vi "LSMcontroller_v56_from here for labview64bit.vi"() -> ()   [LabVIEW 2015] (continued)
                            n1346 = call "displayerrors.vi"() -> ("error IO"=w3777:errorcluster)
                            n1347 = call <vilib>:"General Error Handler.vi"("type of dialog (OK msg:1)"=w3776, "error in (no error)"=w3777) -> ("error out"=w3775:errorcluster)  [unwired: 9 in, 4 out]
                            n1348 = call <vilib>:"Clear Errors.vi"("error in (no error)"=w3775) -> ("error out"=w3774:errorcluster)  [unwired: 5 in, 1 out]
                            n1349 = call "seterrors.vi"("error IO"=w3774) -> ()
                          }
                          frame #8 {
                            w3787 = FALSE ("Value (Signaling)")
                            n1350 = local read "save\ndata"() -> (w3782:bool)
                            n1351 = call "2pparameters.vi"("command"="get") -> ("params out"=w3780:T12)  [unwired: 1 in]
                            n1352 = Unbundle By Name(w3780) -> ("auto OD"=w3778:bool)
                            n1353 = case shown="True" w3782 {
                              tunnel: w3781 -> [_ w3794]
                              frame False {
                              }
                              frame True {
                                n1354 = local read "filename prefix"() -> (w3795:string)
                                n1355 = call "closebinaryfiles.vi"() -> ()  [unwired: 12 in]
                                n1356 = local read "data dir"() -> (w3796:path)
                                n1357 = call "saveparams.vi"("timestamp"=w3794, "filename prefix in"=w3795, "data dir in"=w3796) -> ()  [unwired: 1 in]
                              }
                            }
                            n1358 = case shown="True" w3778 {
                              frame False {
                              }
                              frame True {
                                n1359 = call "configuration.vi"("command"="get") -> ("config out"=w3790:T13)  [unwired: 2 in, 1 out]
                                n1360 = call "2pparameters.vi"("command"="get") -> ("params out"=w3793:T12)  [unwired: 1 in]
                                n1361 = Unbundle By Name(w3790) -> ("point OD"=w3788:u16)
                                n1362 = Unbundle By Name(w3793) -> ("ODfilt"=w3789:u16)
                                n1363 = call "filterwheelcontrol_nothorlabslib.vi"("Current OD filt"=w3788, "New ODfilt"=w3789) -> ()  [unwired: 1 in]
                              }
                            }
                            n1364 = call "reset AO_DO_v3.vi"() -> ()  [unwired: 12 in]
                            n1365 = property on="Start" class="Bool (strict)"("Val(Sgnl)"=w3787) -> ()  [unwired: 2 in, 2 out]
                            n1366 = property on="Start" class="Bool (strict)"("Visible"=TRUE, "DisabledEnum"=T8."Enabled" ("Disabled")) -> ()  [unwired: 2 in, 2 out]
                            n1367 = property on="Stop" class="Bool (strict)"("Val(Sgnl)"=w3787) -> ()  [unwired: 2 in, 2 out]
                            n1368 = property on="Stop" class="Bool (strict)"("Visible"=FALSE, "DisabledEnum"=T8."Disabled" ("Disabled")) -> ()  [unwired: 2 in, 2 out]
                          }
                        }
                      }
                      frame "Line" {
                      }
                      frame "Resonant Ellipse", "freeform contour" {
                        n1369 = stacked-sequence {
                          seq-local: [w3811 _ _ _ _ _ _ _ _ _ _] -> [_ _ w4656 _ _ w4669 w4736 _ _ w5096 _]
                          seq-local: [w3810 _ _ _ _ _ _ _ _ _ _] -> [_ _ _ _ _ _ _ _ w4783 _ _]
                          seq-local: [w3809 _ _ _ _ _ _ _ _ _ _] -> [_ _ _ _ _ _ _ _ w4782 _ _]
                          seq-local: [w3808 _ _ _ _ _ _ _ _ _ _] -> [_ _ _ _ _ _ _ _ w4785 _ _]
                          seq-local: [w3807 _ _ _ _ _ _ _ _ _ _] -> [_ _ _ _ _ _ _ _ w4781 _ _]
                          seq-local: [w3806 _ _ _ _ _ _ _ _ _ _] -> [_ _ _ _ _ _ _ _ w4780 _ _]
                          seq-local: [w3805 _ _ _ _ _ _ _ _ _ _] -> [_ _ _ _ _ _ _ _ w4784 _ _]
                          seq-local: [w3804 _ _ _ _ _ _ _ _ _ _] -> [_ _ _ _ _ _ _ _ w4779 _ _]
                          seq-local: [w3803 _ _ _ _ _ _ _ _ _ _] -> [_ _ _ _ _ _ _ _ w4778 _ _]
                          seq-local: [w3802 _ _ _ _ _ _ _ _ _ _] -> [_ _ _ _ _ _ _ _ w4773 _ _]
                          seq-local: [w3801 _ _ _ _ _ _ _ _ _ _] -> [_ _ _ _ _ _ _ _ w4772 _ _]
                          seq-local: [w3800 _ _ _ _ _ _ _ _ _ _] -> [_ _ _ _ _ _ _ _ w4777 _ _]
                          seq-local: [w3799 _ _ _ _ _ _ _ _ _ _] -> [_ _ _ _ _ _ _ _ w4776 _ _]
                          seq-local: [w3798 _ _ _ _ _ _ _ _ _ _] -> [_ _ _ _ _ _ _ _ w4775 _ _]
                          seq-local: [w3797 _ _ _ _ _ _ _ _ _ _] -> [_ _ _ _ _ _ _ _ w4774 _ _]
                          frame #0 {
                            n1370 = local read "save\ndata"() -> (w3812:bool)
                            n1371 = Get Date/Time In Seconds() -> (seconds since 1Jan1904=w3813:timestamp)
                            n1372 = case shown="False" w3812 {
                              tunnel: w3813 -> [w3814 w3816]
                              tunnel: [w3814 w3815] -> w3811
                              frame False {
                              }
                              frame True {
                                n1373 = call "createdatafolder.vi"("timestamp in"=w3816) -> ("current data path"=w3817:path, "timestamp out"=w3815:timestamp)
                                n1374 = local write "data dir"(w3817) -> ()
                              }
                            }
                            n1375 = stacked-sequence {
                              tunnel: w3811 -> [w3823 _ _ _ _ _ _ _ _]
                              tunnel: [_ _ _ _ _ _ w3961 _ _] -> w3810
                              tunnel: [_ _ _ _ _ _ w3960 _ _] -> w3809
                              tunnel: [_ _ _ _ _ _ w3959 _ _] -> w3808
                              tunnel: [_ _ _ _ _ _ w3958 _ _] -> w3807
                              tunnel: [_ _ _ _ _ _ w3957 _ _] -> w3806
                              tunnel: [_ _ _ _ _ _ w3956 _ _] -> w3805
                              tunnel: [_ _ _ _ _ _ w3955 _ _] -> w3804
                              tunnel: [_ _ _ _ _ _ w3954 _ _] -> w3803
                              tunnel: [_ _ _ _ _ _ w3953 _ _] -> w3802
                              tunnel: [_ _ _ _ _ _ w3952 _ _] -> w3801
                              tunnel: [_ _ _ _ _ _ w3951 _ _] -> w3800
                              tunnel: [_ _ _ _ _ _ w3950 _ _] -> w3799
                              tunnel: [_ _ _ _ _ _ w3949 _ _] -> w3798
                              tunnel: [_ _ _ _ _ _ w3948 _ _] -> w3797
                              frame #0 {
                                n1376 = local write "graphtab"(T6."timetrace" ("graphtab")) -> ()
                                n1377 = local read "AI channels"() -> (w3827:i32[])
                                n1378 = local read "CI channels"() -> (w3828:i32[])
                                n1379 = property on="Stop" class="Bool (strict)"("Visible"=TRUE, "DisabledEnum"=T8."Enabled" ("Disabled")) -> ()  [unwired: 2 in, 2 out]
                                n1380 = property on="Start" class="Bool (strict)"("Visible"=FALSE, "DisabledEnum"=T8."Disabled and Grayed Out" ("Disabled")) -> ()  [unwired: 2 in, 2 out]
                                n1381 = Format Date/Time String(time format string (%c)="%Y%m%d", seconds (now)=w3823) -> (date/time string=w3822:string)  [unwired: 1 in]
                                n1382 = Format Date/Time String(time format string (%c)="%H%M%S", seconds (now)=w3823) -> (date/time string=w3821:string)  [unwired: 1 in]
                                n1383 = call "2pparameters.vi"("command"="get") -> ("params out"=w3830:T12)  [unwired: 1 in]
                                n1384 = Bundle By Name(cluster=w3830, "aAI"=w3827, "aCI"=w3828, "type"="Timetrace", "date"=w3822, "time"=w3821) -> (w3829:T12)
                                n1385 = call "X-array-databuffer.vi"("command"=enum16{"get", "set", "clear", "append"}."clear") -> ()  [unwired: 3 in, 2 out]
                                n1386 = call "Y-array-databuffer.vi"("command"=enum16{"get", "set", "clear", "append"}."clear") -> ()  [unwired: 3 in, 2 out]
                                n1387 = call "2pparameters.vi"("Params in"=w3829, "command"="set") -> ()  [unwired: 1 out]
                                n1388 = call "CH1-1D-temp.vi"("command"=enum16{"get", "set", "clear", "append"}."clear") -> ()  [unwired: 3 in, 2 out]
                                n1389 = call "CH2-1D-temp.vi"("command"=enum16{"get", "set", "clear", "append"}."clear") -> ()  [unwired: 3 in, 2 out]
                                n1390 = call "allAI-temp.vi"("command"=enum16{"get", "set", "clear", "append"}."clear") -> ()  [unwired: 3 in, 2 out]
                              }
                              frame #1 {
                                n1391 = call "configuration.vi"("command"="get") -> ("config out"=w3847:T13)  [unwired: 2 in, 1 out]
                                n1392 = Unbundle By Name(w3847) -> ("CI names"=w3848:string[], "AI names"=w3849:string[])
                                n1393 = call "2pparameters.vi"("command"="get") -> ("params out"=w3843:T12)  [unwired: 1 in]
                                n1394 = Unbundle By Name(w3843) -> ("aCI"=w3844:i32[], "aAI"=w3845:i32[])
                                n1395 = for {
                                tunnel: w3844 -> [w3859] mode=indexing
                                tunnel: w3848 -> [w3860]
                                tunnel: [w3858] -> w3850 mode=indexing
                                n1396 = Index Array(array=w3860, index=w3859) -> (element=w3858:string)
                                }
                                n1397 = for {
                                tunnel: w3845 -> [w3856] mode=indexing
                                tunnel: w3849 -> [w3857]
                                tunnel: [w3855] -> w3851 mode=indexing
                                n1398 = Index Array(array=w3857, index=w3856) -> (element=w3855:string)
                                }
                                n1399 = Build Array (concatenate)(w3850, w3851) -> (w3841:string[])
                                n1400 = for {
                                tunnel: w3841 -> [w3853] mode=indexing
                                tunnel: [w3852] -> w3840 mode=indexing
                                i -> [w3854]
                                n1401 = Bundle("String"=w3853, w3854) -> (w3852:cluster{"String":string, i32})  [unwired: 1 in]
                                }
                                n1402 = property on="graph1list" class="Ring (strict)"("StringsAndValues[]"=w3840) -> ()  [unwired: 2 in, 2 out]
                                n1403 = property on="graph2list" class="Ring (strict)"("StringsAndValues[]"=w3840) -> ()  [unwired: 2 in, 2 out]
                              }
                              frame #2 {
                                n1404 = call "2pparameters.vi"("command"="get") -> ("params out"=w3863:T12)  [unwired: 1 in]
                                n1405 = Unbundle By Name(w3863) -> ("auto OD"=w3861:bool, "autoshutter"=w3864:bool)
                                n1406 = case shown="True" w3861 {
                                frame False {
                                }
                                frame True {
                                n1407 = call "configuration.vi"("command"="get") -> ("config out"=w3867:T13)  [unwired: 2 in, 1 out]
                                n1408 = Unbundle By Name(w3867) -> ("contour OD"=w3868:u16)
                                n1409 = local read "ODfilt"() -> (w3865:u16)
                                n1410 = call "filterwheelcontrol_nothorlabslib.vi"("Current OD filt"=w3865, "New ODfilt"=w3868) -> ()  [unwired: 1 in]
                                }
                                }
                                n1411 = case shown="True" w3864 {
                                frame False {
                                }
                                frame True {
                                n1412 = call "shuttercontrol.vi"("command"="close") -> ()  [unwired: 1 in, 1 out]
                                }
                                }
                              }
                              frame #3 {
                                n1413 = local read "Vy-min draw"() -> (w3877:dbl)
                                n1414 = local read "Vy-max draw"() -> (w3876:dbl)
                                n1415 = local read "Vx-min draw"() -> (w3879:dbl)
                                n1416 = local read "Vx-max draw"() -> (w3878:dbl)
                                n1417 = local read "xpixels ref"() -> (w3875:i32)
                                n1418 = local read "ypixels ref"() -> (w3874:i32)
                                n1419 = local read "ROI Type"() -> (w3873:u16)
                                n1420 = local read "srateAODOtt"() -> (w3896:dbl)
                                n1421 = local read "# of frames"() -> (w3901:i32)
                                n1422 = local read "refreshtime"() -> (w3893:dbl)
                                n1423 = local read "Pel"() -> (w3872:dbl)
                                n1424 = local read "bin"() -> (w3899:dbl)
                                n1425 = local read "Override AI buffer"() -> (w3870:bool)
                                n1426 = local read "finite samples"() -> (w3908:bool)
                                n1427 = local read "srateAODOtt"() -> (w3895:dbl)
                                n1428 = local read "srateAODOtt"() -> (w3902:dbl)
                                n1429 = local read "continuous"() -> (w3907:bool)
                                n1430 = local read "Angle ref"() -> (w3880:dbl)
                                n1431 = local read "wavdet"() -> (w3909:bool)
                                n1432 = local read "Vx-ref"() -> (w3904:dbl)
                                n1433 = local read "Vy-ref"() -> (w3906:dbl)
                                n1434 = local read "avpp"() -> (w3905:i32)
                                n1435 = call "tt_timeandsamples.vi"("bin"=w3899, "refreshtime"=w3893, "srateAODOtt"=w3896, "tot#ofsamples"=w3901) -> ("refreshrate"=w3897:dbl, "refreshbuffer"=w3898:i32, "timetracecycles"=w3903:i32)  [unwired: 5 in]
                                n1436 = local read "bin"() -> (w3900:dbl)
                                n1437 = call "2pparameters.vi"("command"="get") -> ("params out"=w3912:T12)  [unwired: 1 in]
                                n1438 = Bundle By Name(cluster=w3912, "Drawing Mode"=w3873, "measpoints"=w3901, "tt_cycles"=w3903, "refreshbuffer"=w3898, "refreshrate"=w3897, "Vx-ref"=w3904, "Vy-ref"=w3906, "srate"=w3895, "finite"=w3908, "cont"=w3907, "wavdet"=w3909, "avpp"=w3905, "srateAODO"=w3902, "bufferAI"=w3898, "bin"=w3900, "Angle Img"=w3880, "Vxminref"=w3879, "Vxmaxref"=w3878, "Vyminref"=w3877, "Vymaxref"=w3876, "Xpixels Img"=w3875, "Ypixels Img"=w3874, "Pel"=w3872, "Vz-reset"=0.0, "AIoverride"=w3870) -> (w3910:T12)
                                n1439 = Reciprocal(x=w3897) -> (1/x=w3894:dbl)
                                n1440 = local write "refreshtime"(w3894) -> ()
                                n1441 = call "2pparameters.vi"("Params in"=w3910, "command"="set") -> ()  [unwired: 1 out]
                                n1442 = local read "Voltage Clamp"() -> (w3887:bool)
                                n1443 = local read "Current Clamp"() -> (w3888:bool)
                                n1444 = local read "Vholding (mV)"() -> (w3882:sgl)
                                n1445 = local read "CC_ICgain"() -> (w3886:dbl)
                                n1446 = local read "OCgain"() -> (w3883:sgl)
                                n1447 = local read "holdon"() -> (w3881:bool)
                                n1448 = call "patchparameters.vi"("command"="get") -> ("Params out"=w3890:T15)  [unwired: 1 in]
                                n1449 = Bundle By Name(cluster=w3890, "VC"=w3887, "CC"=w3888, "CC_icg (pA/mv)"=w3886, "VC_icg (mV/mV)"=10.0, "OCG (mV/pA)"=w3883, "OVG (mV/mV)"=0.1, "Vhold (mV)"=w3882, "holdon"=w3881) -> (w3889:T15)
                                n1450 = call "patchparameters.vi"("Params in"=w3889, "command"="set") -> ()  [unwired: 1 out]
                              }
                              frame #4 {
                                n1451 = call "2pparameters.vi"("command"="get") -> ("params out"=w3928:T12)  [unwired: 1 in]
                                n1452 = Unbundle By Name(w3928) -> ("srateAODO"=w3929:sgl, "Angle Img"=w3930:dbl, "Angle draw"=w3931:dbl, "Vxmaxref"=w3932:dbl, "Vxminref"=w3933:dbl, "Xpixels Img"=w3934:i32, "Ypixels Img"=w3935:i32, "Vymaxref"=w3936:dbl, "Vxminref"=w3937:dbl, "Drawing Mode"=w3938:u16, "Pel"=w3939:sgl)
                                n1453 = Add(x=w3930, y=w3931) -> (x+y=w3914:dbl)
                                n1454 = call "ROI-databuffer.vi"("command"=enum16{"get", "set", "clear", "append"}."get") -> ("array out"=w3922:cluster{"x":sgl, "y":sgl}[])  [unwired: 4 in]
                                n1455 = call "ScanningWaveform_v4.vi"("Vy-min"=w3937, "Vy-max"=w3936, "yPixels/tPixels"=w3935, "xPixels/rPixels"=w3934, "Vx-min"=w3933, "Vx-max"=w3932, "Drawing Mode"=w3938, "Angle"=w3914, "AOrate"=w3929, "Points"=w3922, "points in ellipse"=w3939) -> ("numPixels"=w3915:dbl, "Y-WaveArray"=w3916:dbl[], "P"=w3921:dbl, "X-WaveArray"=w3917:dbl[])  [unwired: 5 in]
                                n1456 = call "Y-array-databuffer.vi"("array in"=w3916, "command"=enum16{"get", "set", "clear", "append"}."set") -> ()  [unwired: 2 in, 2 out]
                                n1457 = call "X-array-databuffer.vi"("array in"=w3917, "command"=enum16{"get", "set", "clear", "append"}."set") -> ()  [unwired: 2 in, 2 out]
                                n1458 = call "2pparameters.vi"("command"="get") -> ("params out"=w3926:T12)  [unwired: 1 in]
                                n1459 = Bundle By Name(cluster=w3926, "P"=w3921, "sAOxy"=w3915, "Pel"=w3915) -> (w3918:T12)
                                n1460 = call "2pparameters.vi"("Params in"=w3918, "command"="set") -> ()  [unwired: 1 out]
                              }
                              frame #5 {
                                n1461 = call "X-array-databuffer.vi"("command"=enum16{"get", "set", "clear", "append"}."get") -> ("array out"=w3942:dbl[])  [unwired: 3 in, 1 out]
                                n1462 = call "Y-array-databuffer.vi"("command"=enum16{"get", "set", "clear", "append"}."get") -> ("array out"=w3945:dbl[])  [unwired: 3 in, 1 out]
                                n1463 = Index Array(array=w3942, index=0) -> (element=w3941:dbl)
                                n1464 = Index Array(array=w3945, index=0) -> (element=w3940:dbl)
                                n1465 = call "setposition.vi"("Vy"=w3940, "Vx"=w3941) -> ()  [unwired: 1 in]
                              }
                              frame #6 {
                                # "rem2Ps"
                                # "A2Ps"
                                # "Al"
                                # "Rl"
                                n1466 = stacked-sequence {
                                seq-local: [w3966 _ _ _ _ _ _ _ _ _ _] -> [_ w4078 _ w4139 _ w4225 _ _ _ _ _]
                                seq-local: [w3967 _ _ _ _ _ _ _ _ _ _] -> [_ w4079 w4089 _ w4194 _ _ _ _ _ _]
                                seq-local: [_ _ w4088 _ _ _ _ _ _ _ _] -> [_ _ _ _ w4188 _ _ _ _ _ _]
                                seq-local: [_ _ _ w4138 _ _ _ _ _ _ _] -> [_ _ _ _ _ w4224 _ _ _ _ _]
                                seq-local: [w3963 _ _ _ _ _ _ _ _ _ _] -> [_ w4075 _ _ _ _ _ _ w4410 w4478 _]
                                seq-local: [w3962 _ _ _ _ _ _ _ _ _ _] -> [_ w4074 _ _ _ _ _ _ w4411 w4479 _]
                                seq-local: [w3969 _ _ _ _ _ _ _ _ _ _] -> [_ _ _ _ _ _ w4263 _ w4409 w4477 _]
                                seq-local: [w3965 _ _ _ _ _ _ _ _ _ _] -> [_ w4073 _ _ _ _ w4262 w4330 _ _ _]
                                seq-local: [w3964 _ _ _ _ _ _ _ _ _ _] -> [_ w4072 _ _ _ _ w4261 w4329 _ _ _]
                                seq-local: [w3968 _ _ _ _ _ _ _ _ _ _] -> [_ _ _ _ _ _ w4260 w4328 _ _ _]
                                tunnel: [_ _ w4087 _ _ _ _ _ _ _ _] -> w3960
                                tunnel: [_ _ w4086 _ _ _ _ _ _ _ _] -> w3961
                                tunnel: [w3967 _ _ _ _ _ _ _ _ _ _] -> w3959
                                tunnel: [w3966 _ _ _ _ _ _ _ _ _ _] -> w3956
                                tunnel: [_ _ _ w4137 _ _ _ _ _ _ _] -> w3957
                                tunnel: [_ _ _ w4136 _ _ _ _ _ _ _] -> w3958
                                tunnel: [w3965 _ _ _ _ _ _ _ _ _ _] -> w3951
                                tunnel: [w3964 _ _ _ _ _ _ _ _ _ _] -> w3950
                                tunnel: [_ _ _ _ _ _ w4259 _ _ _ _] -> w3949
                                tunnel: [_ _ _ _ _ _ _ w4327 _ _ _] -> w3948
                                tunnel: [w3963 _ _ _ _ _ _ _ _ _ _] -> w3952
                                tunnel: [w3962 _ _ _ _ _ _ _ _ _ _] -> w3953
                                tunnel: [_ _ _ _ _ _ _ _ w4408 _ _] -> w3954
                                tunnel: [_ _ _ _ _ _ _ _ _ w4476 _] -> w3955
                                frame #0 {
                                # "for a next version, give ome thought to\nthe possibilit of intermittently updating the\nwaveforms. it will have to be a calculation\nbased on speed of CPU and program on the one hand\nand length of measurement on the other. but then it should be possible, in principle, to \nupdate the waveform on the fly and that way cut up a longer measurement in smaller parts."
                                n1467 = stacked-sequence {
                                tunnel: [w3970 _ _ _] -> w3967
                                tunnel: [_ w3982 _ _] -> w3966
                                tunnel: [_ _ _ w4039] -> w3962
                                tunnel: [_ _ _ w4038] -> w3963
                                tunnel: [_ _ _ w4037] -> w3969
                                tunnel: [_ _ w3997 _] -> w3965
                                tunnel: [_ _ w3996 _] -> w3964
                                tunnel: [_ _ w3995 _] -> w3968
                                frame #0 {
                                n1468 = call "configuration.vi"("command"="get") -> ("config out"=w3972:T13)  [unwired: 2 in, 1 out]
                                n1469 = Unbundle By Name(w3972) -> ("Voltage to Xgalvo"=w3971:i32)
                                n1470 = call "2pparameters.vi"("command"="get") -> ("params out"=w3976:T12)  [unwired: 1 in]
                                n1471 = in-place {
                                in-place-border: w3971 -> [w3981]
                                in-place-border: [w3978] -> w3970
                                n1472 = in-place-cluster #23(w3976) -> ("aAO"=w3980:u32[])
                                n1473 = call "add channel to active arrayv2.vi"("line array in"=w3980, "line to add"=w3981) -> ("line array out"=w3979:u32[], "addition"=w3978:bool)  [unwired: 1 out]
                                n1474 = in-place-cluster #23("aAO"=w3979) -> (w3974:T12)
                                }
                                n1475 = call "2pparameters.vi"("Params in"=w3974, "command"="set") -> ()  [unwired: 1 out]
                                }
                                frame #1 {
                                n1476 = call "configuration.vi"("command"="get") -> ("config out"=w3984:T13)  [unwired: 2 in, 1 out]
                                n1477 = Unbundle By Name(w3984) -> ("Voltage to Ygalvo"=w3983:i32)
                                n1478 = call "2pparameters.vi"("command"="get") -> ("params out"=w3988:T12)  [unwired: 1 in]
                                n1479 = in-place {
                                in-place-border: w3983 -> [w3993]
                                in-place-border: [w3990] -> w3982
                                n1480 = in-place-cluster #24(w3988) -> ("aAO"=w3992:u32[])
                                n1481 = call "add channel to active arrayv2.vi"("line array in"=w3992, "line to add"=w3993) -> ("line array out"=w3991:u32[], "addition"=w3990:bool)  [unwired: 1 out]
                                n1482 = in-place-cluster #24("aAO"=w3991) -> (w3986:T12)
                                }
                                n1483 = call "2pparameters.vi"("Params in"=w3986, "command"="set") -> ()  [unwired: 1 out]
                                }
                                frame #2 {
                                n1484 = call "2pparameters.vi"("command"="get") -> ("params out"=w3999:T12)  [unwired: 1 in]
                                n1485 = Unbundle By Name(w3999) -> ("autoshutter"=w3998:bool, "wavdet"=w3994:bool)
                                n1486 = case shown="False" w3998 {
                                tunnel: [w4004 w4024] -> w3997
                                tunnel: [w4003 FALSE ("removal")] -> w3996
                                tunnel: [w4002 w4022] -> w3995
                                tunnel: w3994 -> [w4001 _]
                                frame False {
                                n1487 = case shown="False" w4001 {
                                tunnel: [FALSE ("addition") FALSE ("addition")] -> w4004
                                tunnel: [w4006 FALSE ("removal")] -> w4003
                                tunnel: [w4005 _] -> w4002
                                frame False {
                                n1488 = call "configuration.vi"("command"="get") -> ("config out"=w4012:T13)  [unwired: 2 in, 1 out]
                                n1489 = Unbundle By Name(w4012) -> ("2P shutter"=w4009:i32)
                                n1490 = call "2pparameters.vi"("command"="get") -> ("params out"=w4010:T12)  [unwired: 1 in]
                                n1491 = in-place {
                                in-place-border: w4009 -> [w4019]
                                in-place-border: [w4016] -> w4006
                                in-place-border: [w4015] -> w4005
                                n1492 = in-place-cluster #25(w4010) -> ("aDO"=w4018:u32[])
                                n1493 = call "remove channel from active arrayv2.vi"("line array in"=w4018, "line to remove"=w4019) -> ("line array out"=w4017:u32[], "removal"=w4016:bool, "index"=w4015:i32)
                                n1494 = in-place-cluster #25("aDO"=w4017) -> (w4007:T12)
                                }
                                n1495 = call "2pparameters.vi"("Params in"=w4007, "command"="set") -> ()  [unwired: 1 out]
                                }
                                frame True {
                                }
                                }
                                }
                                frame True {
                                n1496 = call "configuration.vi"("command"="get") -> ("config out"=w4026:T13)  [unwired: 2 in, 1 out]
                                n1497 = call "2pparameters.vi"("command"="get") -> ("params out"=w4030:T12)  [unwired: 1 in]
                                n1498 = Unbundle By Name(w4026) -> ("2P shutter"=w4025:i32)
                                n1499 = in-place {
                                in-place-border: w4025 -> [w4036]
                                in-place-border: [w4033] -> w4024
                                in-place-border: [w4032] -> w4022
                                n1500 = in-place-cluster #26(w4030) -> ("aDO"=w4035:u32[])
                                n1501 = call "add channel to active arrayv2.vi"("line array in"=w4035, "line to add"=w4036) -> ("line array out"=w4034:u32[], "addition"=w4033:bool, "index"=w4032:i32)
                                n1502 = in-place-cluster #26("aDO"=w4034) -> (w4028:T12)
                                }
                                n1503 = call "2pparameters.vi"("Params in"=w4028, "command"="set") -> ()  [unwired: 1 out]
                                }
                                }
                                }
                                frame #3 {
                                n1504 = local read "Measurement"() -> (w4040:T5)
                                n1505 = To Unsigned Long Integer(number=w4040) -> (unsigned 32bit integer=w4041:u32)
                                n1506 = case shown="5..7" w4041 {
                                tunnel: [FALSE ("addition") w4059] -> w4039
                                tunnel: [w4044 FALSE ("removal")] -> w4038
                                tunnel: [w4042 w4057] -> w4037
                                frame 0..4, Default {
                                n1507 = call "configuration.vi"("command"="get") -> ("config out"=w4050:T13)  [unwired: 2 in, 1 out]
                                n1508 = Unbundle By Name(w4050) -> ("LT timestamp"=w4047:u32)
                                n1509 = call "2pparameters.vi"("command"="get") -> ("params out"=w4048:T12)  [unwired: 1 in]
                                n1510 = in-place {
                                in-place-border: w4047 -> [w4056]
                                in-place-border: [w4053] -> w4044
                                in-place-border: [w4052] -> w4042
                                n1511 = in-place-cluster #27(w4048) -> ("aDO"=w4055:u32[])
                                n1512 = call "remove channel from active arrayv2.vi"("line array in"=w4055, "line to remove"=w4056) -> ("line array out"=w4054:u32[], "removal"=w4053:bool, "index"=w4052:i32)
                                n1513 = in-place-cluster #27("aDO"=w4054) -> (w4045:T12)
                                }
                                n1514 = call "2pparameters.vi"("Params in"=w4045, "command"="set") -> ()  [unwired: 1 out]
                                }
                                frame 5..7 {
                                n1515 = call "configuration.vi"("command"="get") -> ("config out"=w4065:T13)  [unwired: 2 in, 1 out]
                                n1516 = Unbundle By Name(w4065) -> ("LT timestamp"=w4062:u32)
                                n1517 = call "2pparameters.vi"("command"="get") -> ("params out"=w4063:T12)  [unwired: 1 in]
                                n1518 = in-place {
                                in-place-border: w4062 -> [w4071]
                                in-place-border: [w4068] -> w4059
                                in-place-border: [w4067] -> w4057
                                n1519 = in-place-cluster #28(w4063) -> ("aDO"=w4070:u32[])
                                n1520 = call "add channel to active arrayv2.vi"("line array in"=w4070, "line to add"=w4071) -> ("line array out"=w4069:u32[], "addition"=w4068:bool, "index"=w4067:i32)
                                n1521 = in-place-cluster #28("aDO"=w4069) -> (w4060:T12)
                                }
                                n1522 = call "2pparameters.vi"("Params in"=w4060, "command"="set") -> ()  [unwired: 1 out]
                                }
                                }
                                }
                                }
                                }
                                frame #1 {
                                n1523 = Or(x=w4078, y=w4079) -> (x .or. y?=w4077:bool)
                                n1524 = case shown="True" w4077 {
                                frame False {
                                }
                                frame True {
                                # "update GUI"
                                n1525 = call "Used AO lines.vi"() -> ("used AO names"=w4083:string[], "used AO lines"=w4085:tag[])  [unwired: 2 in]
                                n1526 = control-ref of="Analog Lines Plot"() -> (w4084:refnum<vi>)
                                n1527 = local write "Analog Used Lines"(w4085) -> ()
                                n1528 = local write "Analog Used Names"(w4083) -> ()
                                n1529 = call "prepAOWaveplot.vi"("WaveformGraph in"=w4084, "Analog Used Names"=w4083) -> ()  [unwired: 1 in]
                                }
                                }
                                n1530 = Compound Arithmetic op=OR(w4075, w4074, w4073, w4072) -> (w4076:bool)
                                n1531 = case shown="True" w4076 {
                                frame False {
                                }
                                frame True {
                                n1532 = control-ref of="Digital Lines Plot"() -> (w4080:refnum<vi>)
                                n1533 = call "Used DO lines.vi"() -> ("used DO names"=w4081:string[], "used DO lines"=w4082:tag[])  [unwired: 2 in]
                                n1534 = local write "Digital Used Lines"(w4082) -> ()
                                n1535 = local write "Digital Used Names"(w4081) -> ()
                                n1536 = call "prepDOWaveplot.vi"("DigitalGraph in"=w4080, "used DO names"=w4081) -> ()  [unwired: 1 in]
                                }
                                }
                                }
                                frame #2 {
                                n1537 = case shown="False" w4089 {
                                tunnel: [w4092 w4118] -> w4088
                                tunnel: [w4091 w4116] -> w4087
                                tunnel: [w4090 _] -> w4086
                                frame False {
                                n1538 = stacked-sequence {
                                seq-local: [w4094 _] -> [_ w4109]
                                tunnel: [w4094 _] -> w4092
                                tunnel: [w4097 _] -> w4091
                                tunnel: [w4093 _] -> w4090
                                frame #0 {
                                n1539 = call "configuration.vi"("command"="get") -> ("config out"=w4105:T13)  [unwired: 2 in, 1 out]
                                n1540 = call "waveformparamsv2.vi"("command"="get") -> ("Params out"=w4099:T16)  [unwired: 4 in, 2 out]
                                n1541 = Unbundle By Name(w4105) -> ("Voltage to Xgalvo"=w4106:i32)
                                n1542 = call "2pparameters.vi"("command"="get") -> ("params out"=w4102:T12)  [unwired: 1 in]
                                n1543 = Unbundle By Name(w4099) -> ("AO parameters"=w4098:T17)
                                n1544 = Unbundle By Name(w4102) -> ("aAO"=w4103:u32[])
                                n1545 = call "waveformsAObuffer.vi"("command"="get") -> ("AO wf out"=w4095:waveform(dbl)[])  [unwired: 1 in]
                                n1546 = Search 1D Array(1D array=w4103, element=w4106) -> (index of element=w4094:i32)  [unwired: 1 in]
                                n1547 = Index Array(array=w4095, index=w4094) -> (element=w4093:waveform(dbl))
                                n1548 = Index Array(array=w4098, index=w4094) -> (element=w4097:T18)
                                }
                                frame #1 {
                                w4110 = 0.0 ("Step size (V)")
                                n1549 = local read "Meastab"() -> (w4108:enum32{"X-Y Image", "Linescan", "Timetrace"})
                                n1550 = case shown="\"X-Y Image\", Default" w4108 {
                                tunnel: [w4112 w4113] -> w4107
                                frame "X-Y Image", Default {
                                n1551 = local read "Sampling rate"() -> (w4112:dbl)
                                }
                                frame "Timetrace" {
                                n1552 = local read "srateAODOtt"() -> (w4113:dbl)
                                }
                                }
                                n1553 = call "replace AO XYwfparam.vi"("Baseline (V)"=w4110, "Start amplitude (V)"=w4110, "Cycles"=w4110, "Repeats"=w4110, "index of AO wave"=w4109, "Step size (V)"=w4110, "DC (%)"=w4110, "Sampling frequency (Hz)"=w4107, "Period (ms)"=w4110, "Cycle length (s)"=w4110, "Pulses"=w4110, "padding value"=w4110, "Matlab wave name"=path "xwave") -> ()  [unwired: 3 in]
                                }
                                }
                                }
                                frame True {
                                w4117 = 0.0 ("Repeats")
                                n1554 = local read "Meastab"() -> (w4115:enum32{"X-Y Image", "Linescan", "Timetrace"})
                                n1555 = case shown="\"X-Y Image\", Default" w4115 {
                                tunnel: [w4134 w4135] -> w4114
                                frame "X-Y Image", Default {
                                n1556 = local read "Sampling rate"() -> (w4134:dbl)
                                }
                                frame "Timetrace" {
                                n1557 = local read "srateAODOtt"() -> (w4135:dbl)
                                }
                                }
                                n1558 = call "2pparameters.vi"("command"="get") -> ("params out"=w4120:T12)  [unwired: 1 in]
                                n1559 = call "configuration.vi"("command"="get") -> ("config out"=w4123:T13)  [unwired: 2 in, 1 out]
                                n1560 = call "waveformparamsv2.vi"("command"="get") -> ("Params out"=w4131:T16)  [unwired: 4 in, 2 out]
                                n1561 = Unbundle By Name(w4123) -> ("Voltage to Xgalvo"=w4124:i32)
                                n1562 = Unbundle By Name(w4131) -> ("AO parameters"=w4128:T17)
                                n1563 = Unbundle By Name(w4120) -> ("aAO"=w4121:u32[])
                                n1564 = Search 1D Array(1D array=w4121, element=w4124) -> (index of element=w4118:i32)  [unwired: 1 in]
                                n1565 = Index Array(array=w4128, index=0) -> (element=w4129:T18)
                                n1566 = Bundle By Name(cluster=w4129, "AOtab"=-1.0 ("Repeats"), "Repeats"=w4117, "Cycles"=w4117, "Start amplitude (V)"=w4117, "Baseline (V)"=w4117, "Step size (V)"=w4117, "DC (%)"=w4117, "Sampling frequency (Hz)"=w4114, "Period (ms)"=w4117, "Offset (V)"=w4117, "Amplitude (V)"=w4117, "Frequency"=w4117, "Tri Repeats"=w4117, "phase shift (ms)"=w4117, "Pulses"=w4117, "Matlab wave file"=path "xwave", "padding value"=w4117) -> (w4116:T18)
                                n1567 = Build Array(w4116) -> (w4126:T17)
                                n1568 = call "waveformparamsv2.vi"("command"="add AO", "add AO"=w4126) -> ()  [unwired: 3 in, 3 out]
                                }
                                }
                                }
                                frame #3 {
                                n1569 = case shown="True" w4139 {
                                tunnel: [w4142 w4168] -> w4138
                                tunnel: [w4141 w4166] -> w4137
                                tunnel: [w4140 _] -> w4136
                                frame False {
                                n1570 = stacked-sequence {
                                seq-local: [w4144 _] -> [_ w4159]
                                tunnel: [w4144 _] -> w4142
                                tunnel: [w4147 _] -> w4141
                                tunnel: [w4143 _] -> w4140
                                frame #0 {
                                n1571 = call "configuration.vi"("command"="get") -> ("config out"=w4155:T13)  [unwired: 2 in, 1 out]
                                n1572 = call "waveformparamsv2.vi"("command"="get") -> ("Params out"=w4149:T16)  [unwired: 4 in, 2 out]
                                n1573 = Unbundle By Name(w4155) -> ("Voltage to Ygalvo"=w4156:i32)
                                n1574 = call "2pparameters.vi"("command"="get") -> ("params out"=w4152:T12)  [unwired: 1 in]
                                n1575 = Unbundle By Name(w4149) -> ("AO parameters"=w4148:T17)
                                n1576 = Unbundle By Name(w4152) -> ("aAO"=w4153:u32[])
                                n1577 = call "waveformsAObuffer.vi"("command"="get") -> ("AO wf out"=w4145:waveform(dbl)[])  [unwired: 1 in]
                                n1578 = Search 1D Array(1D array=w4153, element=w4156) -> (index of element=w4144:i32)  [unwired: 1 in]
                                n1579 = Index Array(array=w4145, index=w4144) -> (element=w4143:waveform(dbl))
                                n1580 = Index Array(array=w4148, index=w4144) -> (element=w4147:T18)
                                }
                                frame #1 {
                                w4160 = 0.0 ("Step size (V)")
                                n1581 = local read "Meastab"() -> (w4158:enum32{"X-Y Image", "Linescan", "Timetrace"})
                                n1582 = case shown="\"X-Y Image\", Default" w4158 {
                                tunnel: [w4162 w4163] -> w4157
                                frame "X-Y Image", Default {
                                n1583 = local read "Sampling rate"() -> (w4162:dbl)
                                }
                                frame "Timetrace" {
                                n1584 = local read "srateAODOtt"() -> (w4163:dbl)
                                }
                                }
                                n1585 = call "replace AO XYwfparam.vi"("Baseline (V)"=w4160, "Start amplitude (V)"=w4160, "Cycles"=w4160, "Repeats"=w4160, "index of AO wave"=w4159, "Step size (V)"=w4160, "DC (%)"=w4160, "Sampling frequency (Hz)"=w4157, "Period (ms)"=w4160, "Cycle length (s)"=w4160, "Pulses"=w4160, "padding value"=w4160, "Matlab wave name"=path "ywave") -> ()  [unwired: 3 in]
                                }
                                }
                                }
                                frame True {
                                w4167 = 0.0 ("Repeats")
                                n1586 = local read "Meastab"() -> (w4165:enum32{"X-Y Image", "Linescan", "Timetrace"})
                                n1587 = case shown="\"X-Y Image\", Default" w4165 {
                                tunnel: [w4184 w4185] -> w4164
                                frame "X-Y Image", Default {
                                n1588 = local read "Sampling rate"() -> (w4184:dbl)
                                }
                                frame "Timetrace" {
                                n1589 = local read "srateAODOtt"() -> (w4185:dbl)
                                }
                                }
                                n1590 = call "2pparameters.vi"("command"="get") -> ("params out"=w4170:T12)  [unwired: 1 in]
                                n1591 = call "configuration.vi"("command"="get") -> ("config out"=w4173:T13)  [unwired: 2 in, 1 out]
                                n1592 = call "waveformparamsv2.vi"("command"="get") -> ("Params out"=w4182:T16)  [unwired: 4 in, 2 out]
                                n1593 = Unbundle By Name(w4173) -> ("Voltage to Ygalvo"=w4174:i32)
                                n1594 = Unbundle By Name(w4182) -> ("AO parameters"=w4179:T17)
                                n1595 = Unbundle By Name(w4170) -> ("aAO"=w4171:u32[])
                                n1596 = Search 1D Array(1D array=w4171, element=w4174) -> (index of element=w4168:i32)  [unwired: 1 in]
                                n1597 = Index Array(array=w4179, index=0) -> (element=w4180:T18)
                                n1598 = Bundle By Name(cluster=w4180, "AOtab"=-1.0 ("Repeats"), "Repeats"=w4167, "Cycles"=w4167, "Start amplitude (V)"=w4167, "Baseline (V)"=w4167, "Step size (V)"=w4167, "DC (%)"=w4167, "Sampling frequency (Hz)"=w4164, "Period (ms)"=w4167, "Offset (V)"=w4167, "Amplitude (V)"=w4167, "Frequency"=w4167, "Tri Repeats"=w4167, "phase shift (ms)"=w4167, "Pulses"=w4167, "Matlab wave file"=path "ywave", "padding value"=w4167) -> (w4166:T18)
                                n1599 = Build Array(w4166) -> (w4177:T17)
                                n1600 = call "waveformparamsv2.vi"("command"="add AO", "add AO"=w4177) -> ()  [unwired: 3 in, 3 out]
                                }
                                }
                                }
                                frame #4 {
                                n1601 = call "2pparameters.vi"("command"="get") -> ("params out"=w4191:T12)  [unwired: 1 in]
                                n1602 = Unbundle By Name(w4191) -> ("wavdet"=w4190:bool, "Pel"=w4187:sgl, "refwfsize"=w4186:dbl, "srateAODO"=w4189:sgl)
                                n1603 = case shown="True" w4190 {
                                tunnel: [w4195 w4205] -> w4193
                                tunnel: w4189 -> [w4196 w4207]
                                tunnel: w4187 -> [_ w4203]
                                tunnel: w4186 -> [_ w4202]
                                frame False {
                                n1604 = call "X-array-databuffer.vi"("command"=enum16{"get", "set", "clear", "append"}."get") -> ("array out"=w4199:dbl[])  [unwired: 3 in, 1 out]
                                n1605 = Reciprocal(x=w4196) -> (1/x=w4197:sgl)
                                n1606 = Bundle By Name("Y"=w4199, "dt"=w4197) -> (w4195:waveform(dbl))  [unwired: 1 in]
                                }
                                frame True {
                                n1607 = To Double Precision Float(number=w4203) -> (double precision float=w4204:dbl)
                                n1608 = Divide(x=w4202, y=w4204) -> (x/y=w4201:dbl)
                                n1609 = Round Toward +Infinity(x=w4201) -> (ceil(x): smallest int >= x=w4200:dbl)
                                n1610 = call "X-array-databuffer.vi"("command"=enum16{"get", "set", "clear", "append"}."get") -> ("array out"=w4209:dbl[])  [unwired: 3 in, 1 out]
                                n1611 = Reciprocal(x=w4207) -> (1/x=w4208:sgl)
                                n1612 = for {
                                N: w4200 -> [_]
                                tunnel: w4209 -> [w4211]
                                tunnel: [w4211] -> w4206 mode=concatenating
                                }
                                n1613 = Bundle By Name("Y"=w4206, "dt"=w4208) -> (w4205:waveform(dbl))  [unwired: 1 in]
                                }
                                }
                                n1614 = case shown="True" w4194 {
                                tunnel: w4193 -> [w4213 w4219]
                                tunnel: w4188 -> [w4214 _]
                                frame False {
                                n1615 = call "waveformsAObuffer.vi"("command"="get") -> ("AO wf out"=w4217:waveform(dbl)[])  [unwired: 1 in]
                                n1616 = property on="refwf" class="Ring (strict)" props=["RingText", "Text"]() -> ()  [unwired: 2 in, 3 out]
                                n1617 = Replace Array Subset(array=w4217, new element=w4213, index=w4214) -> (w4212:waveform(dbl)[])
                                n1618 = call "waveformsAObuffer.vi"("AO wf in"=w4212, "command"="set") -> ()  [unwired: 1 out]
                                }
                                frame True {
                                n1619 = call "waveformsAObuffer.vi"("command"="get") -> ("AO wf out"=w4221:waveform(dbl)[])  [unwired: 1 in]
                                n1620 = Build Array (concatenate)(w4221, w4219) -> (w4218:waveform(dbl)[])
                                n1621 = call "waveformsAObuffer.vi"("AO wf in"=w4218, "command"="set") -> ()  [unwired: 1 out]
                                }
                                }
                                }
                                frame #5 {
                                n1622 = call "2pparameters.vi"("command"="get") -> ("params out"=w4233:T12)  [unwired: 1 in]
                                n1623 = Unbundle By Name(w4233) -> ("wavdet"=w4232:bool, "Pel"=w4230:sgl, "refwfsize"=w4231:dbl, "srateAODO"=w4226:sgl)
                                n1624 = To Double Precision Float(number=w4230) -> (double precision float=w4229:dbl)
                                n1625 = Divide(x=w4231, y=w4229) -> (x/y=w4228:dbl)
                                n1626 = Round Toward +Infinity(x=w4228) -> (ceil(x): smallest int >= x=w4227:dbl)
                                n1627 = case shown="True" w4232 {
                                tunnel: [w4237 w4243] -> w4223
                                tunnel: w4227 -> [_ w4240]
                                tunnel: w4226 -> [w4238 w4245]
                                frame False {
                                n1628 = call "Y-array-databuffer.vi"("command"=enum16{"get", "set", "clear", "append"}."get") -> ("array out"=w4235:dbl[])  [unwired: 3 in, 1 out]
                                n1629 = Reciprocal(x=w4238) -> (1/x=w4239:sgl)
                                n1630 = Bundle By Name("Y"=w4235, "dt"=w4239) -> (w4237:waveform(dbl))  [unwired: 1 in]
                                }
                                frame True {
                                n1631 = call "Y-array-databuffer.vi"("command"=enum16{"get", "set", "clear", "append"}."get") -> ("array out"=w4241:dbl[])  [unwired: 3 in, 1 out]
                                n1632 = Reciprocal(x=w4245) -> (1/x=w4246:sgl)
                                n1633 = for {
                                N: w4240 -> [_]
                                tunnel: w4241 -> [w4247]
                                tunnel: [w4247] -> w4244 mode=concatenating
                                }
                                n1634 = Bundle By Name("Y"=w4244, "dt"=w4246) -> (w4243:waveform(dbl))  [unwired: 1 in]
                                }
                                }
                                n1635 = case shown="False" w4225 {
                                tunnel: w4223 -> [w4250 w4255]
                                tunnel: w4224 -> [w4251 _]
                                frame False {
                                n1636 = call "waveformsAObuffer.vi"("command"="get") -> ("AO wf out"=w4253:waveform(dbl)[])  [unwired: 1 in]
                                n1637 = Replace Array Subset(array=w4253, new element=w4250, index=w4251) -> (w4248:waveform(dbl)[])
                                n1638 = call "waveformsAObuffer.vi"("AO wf in"=w4248, "command"="set") -> ()  [unwired: 1 out]
                                }
                                frame True {
                                n1639 = call "waveformsAObuffer.vi"("command"="get") -> ("AO wf out"=w4257:waveform(dbl)[])  [unwired: 1 in]
                                n1640 = Build Array (concatenate)(w4257, w4255) -> (w4254:waveform(dbl)[])
                                n1641 = call "waveformsAObuffer.vi"("AO wf in"=w4254, "command"="set") -> ()  [unwired: 1 out]
                                }
                                }
                                }
                                frame #6 {
                                n1642 = Build Array(w4262, w4261) -> (w4265:bool[])
                                n1643 = Boolean Array To Number(Boolean array=w4265) -> (number=w4264:u32)
                                n1644 = case shown="1" w4264 {
                                tunnel: w4263 -> [_ _ _ _]
                                tunnel: w4260 -> [_ w4288 _ w4301]
                                tunnel: [_ w4287 _ w4298] -> w4259
                                frame 1 {
                                w4275 = 0.0 ("DOtab")
                                n1645 = call "2pparameters.vi"("command"="get") -> ("params out"=w4272:T12)  [unwired: 1 in]
                                n1646 = call "waveformparamsv2.vi"("command"="get") -> ("Params out"=w4283:T16)  [unwired: 4 in, 2 out]
                                n1647 = Unbundle By Name(w4283) -> ("DO parameters"=w4281:T19)
                                n1648 = Unbundle By Name(w4272) -> ("srate"=w4268:sgl, "Pel"=w4271:sgl)
                                n1649 = To Double Precision Float(number=w4268) -> (double precision float=w4266:dbl)
                                n1650 = To Double Precision Float(number=w4268) -> (double precision float=w4267:dbl)
                                n1651 = To Double Precision Float(number=w4271) -> (double precision float=w4270:dbl)
                                n1652 = Divide(x=w4267, y=w4270) -> (x/y=w4269:dbl)
                                n1653 = Index Array(array=w4281, index=0) -> (element=w4280:T20)
                                n1654 = Bundle By Name(cluster=w4280, "Digital DC (%)"=100.0, "Digital phase"=w4275, "Digital Freq (Hz)"=w4269, "Sampling frequency (Hz)"=w4266, "Digital time offset (s)"=w4275, "padding value"=0.0, "matlab wave file"=path "2Pshutter", "DOtab"=0.0) -> (w4278:T20)
                                n1655 = Build Array(w4278) -> (w4277:T19)
                                n1656 = call "waveformparamsv2.vi"("command"="add DO", "add DO"=w4277) -> ()  [unwired: 3 in, 3 out]
                                }
                                frame 2 {
                                n1657 = call "waveformparamsv2.vi"("command"="get") -> ("Params out"=w4290:T16)  [unwired: 4 in, 2 out]
                                n1658 = in-place {
                                in-place-border: w4288 -> [w4294]
                                in-place-border: [w4293] -> w4287
                                n1659 = in-place-cluster #29(w4290) -> ("DO parameters"=w4296:T19)
                                n1660 = Delete From Array(array=w4296, length=1, index=w4294) -> (deleted portion=w4293:T19, array with subset deleted=w4295:T19)
                                n1661 = in-place-cluster #29("DO parameters"=w4295) -> (w4289:T16)
                                }
                                n1662 = call "waveformparamsv2.vi"("command"="set", "Params in"=w4289) -> ()  [unwired: 3 in, 3 out]
                                }
                                frame 3, Default {
                                }
                                frame 0 {
                                n1663 = call "2pparameters.vi"("command"="get") -> ("params out"=w4303:T12)  [unwired: 1 in]
                                n1664 = Unbundle By Name(w4303) -> ("wavdet"=w4300:bool, "autoshutter"=w4302:bool)
                                n1665 = case shown="True" w4302 {
                                tunnel: w4301 -> [_ w4307]
                                tunnel: w4300 -> [_ w4306]
                                tunnel: [_ w4305] -> w4299
                                frame False {
                                }
                                frame True {
                                n1666 = case shown="False" w4306 {
                                tunnel: w4307 -> [w4309 _]
                                tunnel: [w4308 _] -> w4305
                                frame False {
                                n1667 = stacked-sequence {
                                tunnel: w4309 -> [w4311 w4325]
                                tunnel: [w4310 _] -> w4308
                                frame #0 {
                                n1668 = call "waveformparamsv2.vi"("command"="get") -> ("Params out"=w4313:T16)  [unwired: 4 in, 2 out]
                                n1669 = Unbundle By Name(w4313) -> ("DO parameters"=w4312:T19)
                                n1670 = Index Array(array=w4312, index=w4311) -> (element=w4310:T20)
                                }
                                frame #1 {
                                w4324 = 0.0 ("padding value")
                                n1671 = call "2pparameters.vi"("command"="get") -> ("params out"=w4322:T12)  [unwired: 1 in]
                                n1672 = Unbundle By Name(w4322) -> ("srate"=w4319:sgl, "Pel"=w4321:sgl)
                                n1673 = To Double Precision Float(number=w4319) -> (double precision float=w4317:dbl)
                                n1674 = To Double Precision Float(number=w4319) -> (double precision float=w4318:dbl)
                                n1675 = To Double Precision Float(number=w4321) -> (double precision float=w4320:dbl)
                                n1676 = Divide(x=w4318, y=w4320) -> (x/y=w4316:dbl)
                                n1677 = call "replace DO wf param.vi"("Digital Freq (Hz)"=w4316, "Digital DC (%)"=100.0, "Digital phase"=w4324, "Sampling frequency (Hz)"=w4317, "Digital time offset (s)"=w4324, "index of DO wave"=w4325, "padding value"=w4324, "matlab wave file"=path "2Pshutter" ("matlab wave number")) -> ()  [unwired: 3 in]
                                }
                                }
                                }
                                frame True {
                                }
                                }
                                }
                                }
                                n1678 = Build Array(w4299) -> (w4298:T19)
                                }
                                }
                                }
                                frame #7 {
                                n1679 = Build Array(w4330, w4329) -> (w4332:bool[])
                                n1680 = Boolean Array To Number(Boolean array=w4332) -> (number=w4331:u32)
                                n1681 = case shown="0" w4331 {
                                tunnel: w4328 -> [_ w4374 _ w4381]
                                tunnel: [_ w4373 _ w4379] -> w4327
                                frame 1 {
                                n1682 = call "2pparameters.vi"("command"="get") -> ("params out"=w4339:T12)  [unwired: 1 in]
                                n1683 = Unbundle By Name(w4339) -> ("wavdet"=w4340:bool, "Pel"=w4342:sgl, "refwfsize"=w4343:dbl, "srateAODO"=w4341:sgl)
                                n1684 = call "waveformsDObuffer.vi"("command"="get") -> ("DO wf out"=w4335:digitalwaveform[])  [unwired: 1 in]
                                n1685 = case shown="False" w4340 {
                                tunnel: [w4348 w4358] -> w4337
                                tunnel: w4341 -> [w4353 w4369]
                                tunnel: w4342 -> [w4347 w4362]
                                tunnel: w4343 -> [_ w4366]
                                frame False {
                                w4351 = u16 0 items=["unsigned binary", "offset binary", "2's complement"] ("data format (offset binary)")
                                n1686 = Initialize Array(sgl 1.0, w4347) -> (w4344:sgl[])
                                n1687 = Reciprocal(x=w4353) -> (1/x=w4354:sgl)
                                n1688 = Bundle By Name("Y"=w4344, "dt"=w4354) -> (w4349:waveform(sgl))  [unwired: 1 in]
                                n1689 = call-poly <vilib>:"Analog to Digital.vi"("data format (offset binary)"=w4351, "compress digital (T)"=TRUE, "full-scale range (pk-pk)"=1.0, "resolution (16 bit)"=1, "analog waveform"=w4349) -> ("digital waveform"=w4348:digitalwaveform)  [unwired: 3 in, 3 out]
                                }
                                frame True {
                                w4361 = u16 0 items=["unsigned binary", "offset binary", "2's complement"] ("data format (offset binary)")
                                n1690 = To Double Precision Float(number=w4362) -> (double precision float=w4367:dbl)
                                n1691 = Initialize Array(sgl 1.0, w4362) -> (w4355:sgl[])
                                n1692 = Divide(x=w4366, y=w4367) -> (x/y=w4364:dbl)
                                n1693 = Round Toward +Infinity(x=w4364) -> (ceil(x): smallest int >= x=w4365:dbl)
                                n1694 = for {
                                N: w4365 -> [_]
                                tunnel: w4355 -> [w4371]
                                tunnel: [w4371] -> w4368 mode=concatenating
                                }
                                n1695 = Reciprocal(x=w4369) -> (1/x=w4370:sgl)
                                n1696 = Bundle By Name("Y"=w4368, "dt"=w4370) -> (w4359:waveform(sgl))  [unwired: 1 in]
                                n1697 = call-poly <vilib>:"Analog to Digital.vi"("data format (offset binary)"=w4361, "compress digital (T)"=TRUE, "full-scale range (pk-pk)"=1.0, "resolution (16 bit)"=1, "analog waveform"=w4359) -> ("digital waveform"=w4358:digitalwaveform)  [unwired: 3 in, 3 out]
                                }
                                }
                                n1698 = Build Array (concatenate)(w4335, w4337) -> (w4333:digitalwaveform[])
                                n1699 = call "waveformsDObuffer.vi"("DO wf in"=w4333, "command"="set") -> ()  [unwired: 1 out]
                                }
                                frame 2 {
                                n1700 = call "waveformsDObuffer.vi"("command"="get") -> ("DO wf out"=w4376:digitalwaveform[])  [unwired: 1 in]
                                n1701 = Delete From Array(array=w4376, length=1, index=w4374) -> (deleted portion=w4373:digitalwaveform[], array with subset deleted=w4372:digitalwaveform[])
                                n1702 = call "waveformsDObuffer.vi"("DO wf in"=w4372, "command"="set") -> ()  [unwired: 1 out]
                                }
                                frame 3, Default {
                                }
                                frame 0 {
                                n1703 = call "2pparameters.vi"("command"="get") -> ("params out"=w4383:T12)  [unwired: 1 in]
                                n1704 = Unbundle By Name(w4383) -> ("autoshutter"=w4382:bool, "wavdet"=w4380:bool)
                                n1705 = case shown="True" w4382 {
                                tunnel: w4381 -> [_ w4387]
                                tunnel: w4380 -> [_ w4386]
                                tunnel: [_ w4385] -> w4379
                                frame False {
                                }
                                frame True {
                                n1706 = case shown="False" w4386 {
                                tunnel: w4387 -> [w4391 _]
                                tunnel: [w4389 _] -> w4385
                                frame False {
                                w4398 = u16 0 items=["unsigned binary", "offset binary", "2's complement"] ("data format (offset binary)")
                                n1707 = call "2pparameters.vi"("command"="get") -> ("params out"=w4405:T12)  [unwired: 1 in]
                                n1708 = call "waveformsDObuffer.vi"("command"="get") -> ("DO wf out"=w4392:digitalwaveform[])  [unwired: 1 in]
                                n1709 = Unbundle By Name(w4405) -> ("Pel"=w4407:sgl, "srate"=w4406:sgl)
                                n1710 = Index Array(array=w4392, index=w4391) -> (element=w4390:digitalwaveform)
                                n1711 = Build Array(w4390) -> (w4389:digitalwaveform[])
                                n1712 = Initialize Array(sgl 1.0, w4407) -> (w4393:sgl[])
                                n1713 = Reciprocal(x=w4406) -> (1/x=w4400:sgl)
                                n1714 = Bundle By Name("Y"=w4393, "dt"=w4400) -> (w4396:waveform(sgl))  [unwired: 1 in]
                                n1715 = call-poly <vilib>:"Analog to Digital.vi"("data format (offset binary)"=w4398, "compress digital (T)"=TRUE, "full-scale range (pk-pk)"=1.0, "resolution (16 bit)"=1, "analog waveform"=w4396) -> ("digital waveform"=w4403:digitalwaveform)  [unwired: 3 in, 3 out]
                                n1716 = Replace Array Subset(array=w4392, new element=w4403, index=w4391) -> (w4388:digitalwaveform[])
                                n1717 = call "waveformsDObuffer.vi"("DO wf in"=w4388, "command"="set") -> ()  [unwired: 1 out]
                                }
                                frame True {
                                }
                                }
                                }
                                }
                                }
                                }
                                }
                                frame #8 {
                                n1718 = Build Array(w4411, w4410) -> (w4413:bool[])
                                n1719 = Boolean Array To Number(Boolean array=w4413) -> (number=w4412:u32)
                                n1720 = case shown="0" w4412 {
                                tunnel: w4409 -> [_ w4439 _ w4451]
                                tunnel: [_ w4438 _ w4449] -> w4408
                                frame 1 {
                                w4426 = 0.0 ("DOtab")
                                n1721 = call "2pparameters.vi"("command"="get") -> ("params out"=w4424:T12)  [unwired: 1 in]
                                n1722 = call "waveformparamsv2.vi"("command"="get") -> ("Params out"=w4434:T16)  [unwired: 4 in, 2 out]
                                n1723 = Unbundle By Name(w4434) -> ("DO parameters"=w4432:T19)
                                n1724 = Unbundle By Name(w4424) -> ("srate"=w4421:sgl, "Pel"=w4423:sgl)
                                n1725 = To Double Precision Float(number=w4421) -> (double precision float=w4419:dbl)
                                n1726 = To Double Precision Float(number=w4421) -> (double precision float=w4420:dbl)
                                n1727 = To Double Precision Float(number=w4423) -> (double precision float=w4415:dbl)
                                n1728 = Divide(x=w4420, y=w4415) -> (x/y=w4422:dbl)
